vi "Update Measurement Selection.vi"(8 "error in (no error)":errorcluster, 10 "mouseDown coords":T1, 11 "multicolumnListbox in":refnum<vi>) -> (0 "error out":errorcluster, 3 "multicolumnListbox out":refnum<vi>)   [LabVIEW 2021, in "MeasurementClient Editor.lvlib"]
uses:
  MeasurementClient Editor.lvlib
  <vilib>/Utility/miscctls.llb/LVPoint32TypeDef.ctl
  <vilib>/Utility/miscctls.llb/LVPositionTypeDef.ctl
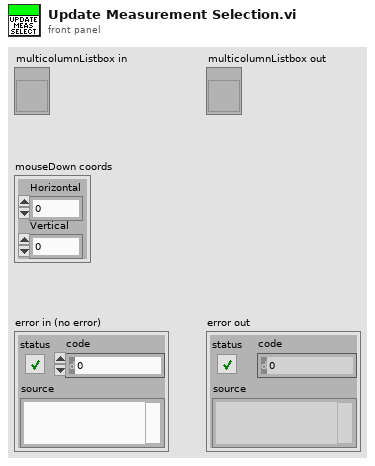
[diagram p1: front panel]
types:
  T1 = typedef "LVPoint32TypeDef.ctl" = cluster{"Horizontal":i32, "Vertical":i32}
  T2 = typedef "LVPositionTypeDef.ctl" = cluster{"Left":i32, "Top":i32}
  T3 = typedef "LVRowAndColumnTypeDef.ctl" = cluster{"Row":i32, "Column":i32}
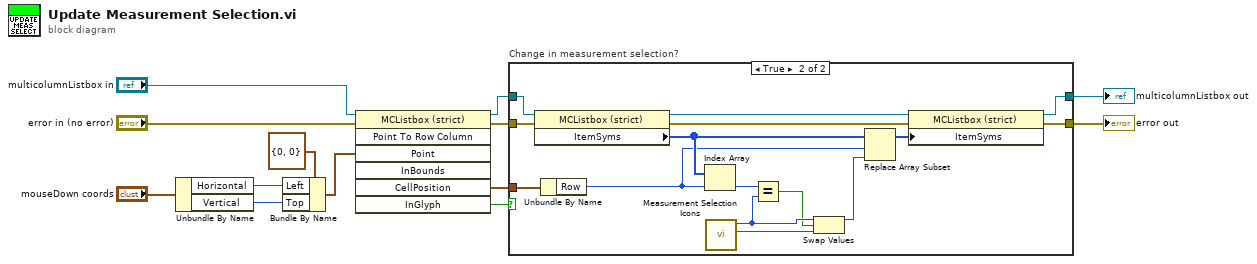
[diagram p0: block diagram]
diagram:
  n1 = Unbundle By Name("mouseDown coords") -> ("Horizontal"=w2:i32, "Vertical"=w1:i32)
  n2 = Bundle By Name(cluster=T2 {"Left"=0, "Top"=0} ("Point"), "Left"=w2, "Top"=w1) -> (w3:T2)
  n3 = invoke class="MCListbox (strict)" method="Point To Row Column"(reference="multicolumnListbox in", error in="error in (no error)", "Point"=w3) -> (reference out=w11:refnum<vi>, error out=w9:errorcluster, "CellPosition"=w10:T3, "InGlyph"=w6:bool)  [unwired: 4 in, 3 out]
  n4 = case "Change in measurement selection?" shown="True" w6 {
    tunnel: w9 -> [w14 w30]
    tunnel: w10 -> [_ w28]
    tunnel: w11 -> [w15 w29]
    tunnel: [w15 w17] -> w12
    tunnel: [w14 w16] -> w13
    frame False {
    }
    frame True {
      n5 = property class="MCListbox (strict)"(reference=w29, error in=w30) -> (reference out=w20:refnum<vi>, error out=w19:errorcluster, "ItemSyms"=w23:i32[])
      n6 = Unbundle By Name(w28) -> ("Row"=w22:i32)
      n7 = Index Array(array=w23, index=w22) -> (element=w25:i32)
      n8 = call "Measurement Selection Icons.vi"() -> ("Checked"=w27:i32, "Unchecked"=w26:i32)  [unwired: 10 in]
      n9 = Equal?(x=w25, y=w26) -> (x = y?=w24:bool)
      n10 = Swap Values(12:w26, 13:w24, 14:w27) -> (1:w21:i32)  [unwired: 1 out]
      n11 = Replace Array Subset(array=w23, new element=w21, index=w22) -> (w18:i32[])
      n12 = property class="MCListbox (strict)"(reference=w20, error in=w19, "ItemSyms"=w18) -> (reference out=w17:refnum<vi>, error out=w16:errorcluster)
    }
  }
  "error out" <- w13
  "multicolumnListbox out" <- w12
